vi "acquire waveform.vi"(0 "Connection ID":refnum<k5>, 5 "Server Stats":T1={"scan rate"=10.0, "# connections"=0, "channel settings"=[]} {"channel settings"."lower input limits" format="%.4f"; "channel settings"."upper input limits" format="%.4f"; "scan rate" format="%.2f"}, 7 "method":T2={"sampling interval"=0.1, "samples to average"=1, "data interval"=0.0, "stream data"=FALSE, "file path"=refnum, "command"={"command"=enum."Idle", "start time (ms)"=0, "Channel Indices"=[], "Scans per Sample"=1}} {"command"."Scans per Sample" min=1; "data interval" format="%.2f"; "samples to average" min=1 step=1; "sampling interval" format="%.2f"}, 11 "data points to acquire":u32=1000 min=1) -> (4 "data array":sgl[][](array[numeric]) format="%.5f", 6 "offset":sgl format="%.5f", 8 "percent CV":sgl format="%.5f")   [LabVIEW 2010]
uses:
  DataServer/command.ctl
  DataServer/command cluster.ctl
  DAC apps/support/method.ctl
  DataServer/Server stats.ctl
panel:
  in  "colors":u32[](array[colorbox])=[16711680, 13311, 52224, 16777215, 16750848, 16738047, 52479, 16776960, 16711680, 13311, 52224, 16777215, 16737792, 16738047, 52479, 16776960]
  out "sample time":dbl format="%.2f"
  out "stop":bool
  in  "State":cluster{"Monitor sample":bool, "Okay":bool}
  out "Scan rate":dbl=10.0
  out "data rate":sgl format="%.4f"
  out "sampling rate":dbl format="%.4f"
  out "chart":sgl[][](graph)
  in  "Monitoring sample":bool
  in  "error":errorcluster={"status"=FALSE, "code"=56, "source"="TCP Read in \u0000TCP read variable.vi->read Volts data fast.vi->Signal Monitor"}
  # "hz"
  # "hz"
  # "hz"
  # "s"
  # "Hz"
  # "s"
  # "s"
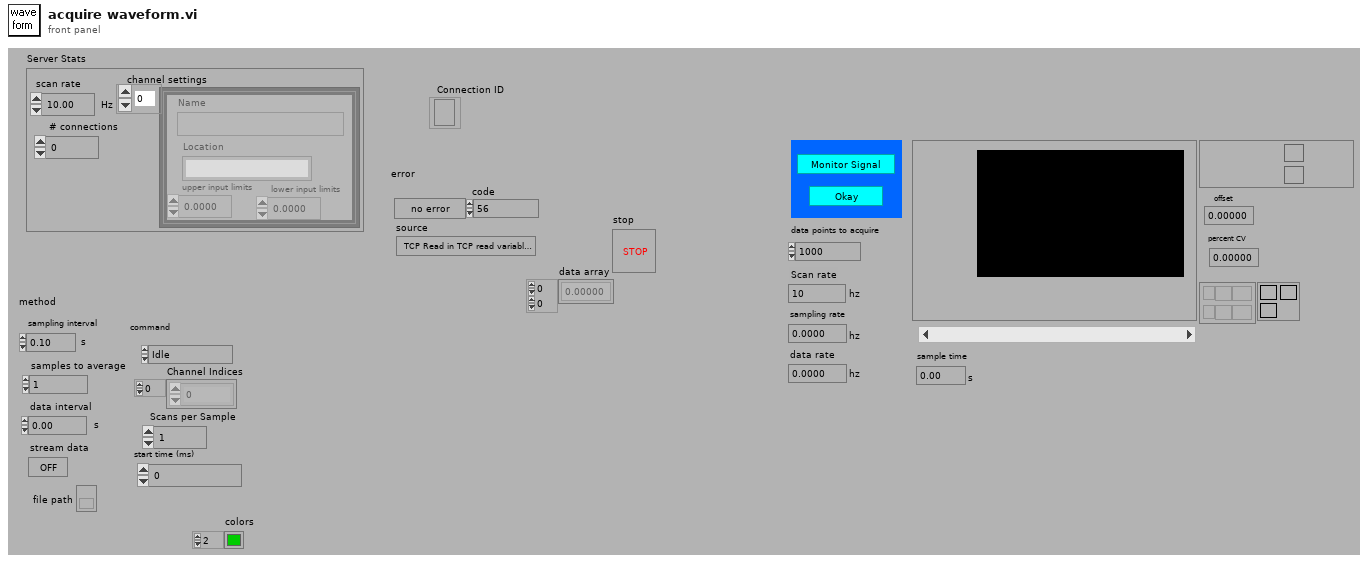
[diagram p1: front panel]
types:
  T1 = typedef "Server stats.ctl" = cluster{"scan rate":dbl, "# connections":i32, "channel settings":cluster{"Name":string, "upper input limits":sgl, "lower input limits":sgl, "Location":string}[]}
  T2 = typedef "method.ctl" = cluster{"sampling interval":sgl, "samples to average":u32, "data interval":sgl, "stream data":bool, "file path":refnum<file>, "command":T3}
  T3 = typedef "command cluster.ctl" = cluster{"command":T4, "start time (ms)":u32, "Channel Indices":i32[], "Scans per Sample":i32}
  T4 = typedef "command.ctl" = enum16{"Idle", "Send Data", "Send 1 Scan", "Logoff"}
  T5 = cluster{"channel":string, "upper input limits":sgl, "lower input limits":sgl, "range":sgl, "polarity":enum16{"no change", "bipolar", "unipolar"}, "gain":sgl, "coupling":enum16{"no change", "DC", "AC", "ground", "internal reference"}, "input mode":enum16{"no change", "differential", "rse", "nrse"}, "scale multiplier":sgl, "scale offset":sgl}[]
  T6 = cluster{"channel":string, "upper input limits":sgl, "lower input limits":sgl, "range":sgl, "polarity":enum16{"no change", "bipolar", "unipolar"}, "gain":sgl, "coupling":enum16{"no change", "DC", "AC", "ground", "internal reference"}, "input mode":enum16{"no change", "differential", "rse", "nrse"}, "scale multiplier":sgl, "scale offset":sgl}
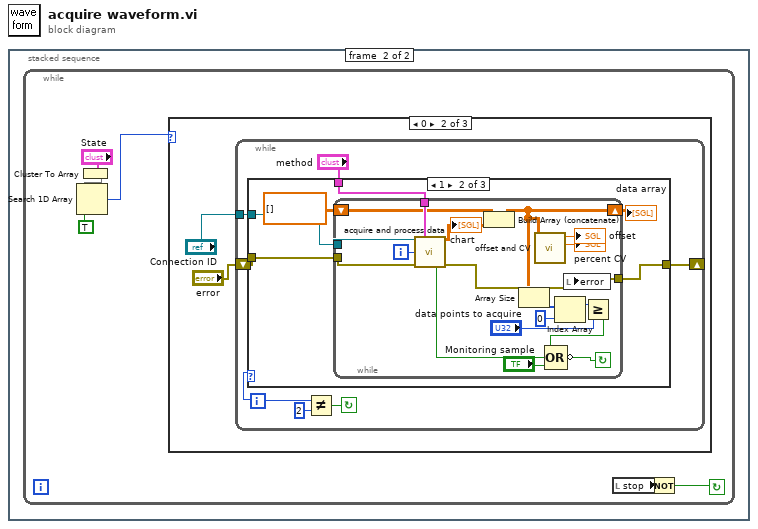
[diagram p0: block diagram]
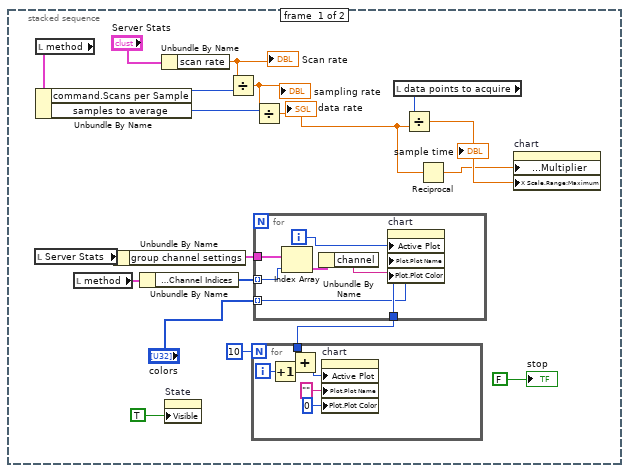
[diagram p2: hidden frame]
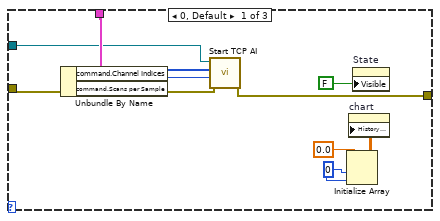
[diagram p4: hidden frame]
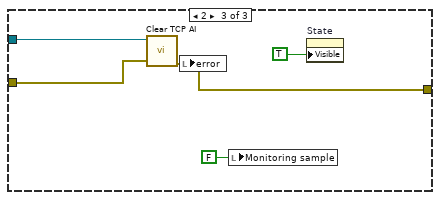
[diagram p5: hidden frame]
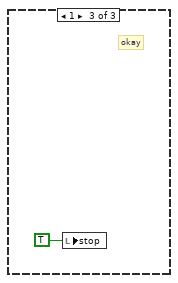
[diagram p6: hidden frame]
diagram:
  n1 = stacked-sequence {
    frame #0 {
      n2 = local read "Server Stats"() -> (w18:T1)
      n3 = local read "method"() -> (w2:T2)
      n4 = Unbundle By Name(w2) -> ("command.Scans per Sample"=w7:i32, "samples to average"=w8:u32)
      n5 = local read "method"() -> (w17:T2)
      n6 = Unbundle By Name(w18) -> ("group channel settings"=w15:T5)
      n7 = Unbundle By Name(w17) -> ("command.Channel Indices"=w16:i32[])
      n8 = Unbundle By Name("Server Stats") -> ("scan rate"=w10:dbl)
      "Scan rate" <- w10
      n9 = property on="State" class="Clust"("Visible"=TRUE ("Write Attribute")) -> ()  [unwired: 2 in, 2 out]
      n10 = Divide(x=w10, y=w7) -> (x/y=w9:dbl)
      "sampling rate" <- w9
      n11 = Divide(x=w9, y=w8) -> (x/y=w4:dbl)
      "data rate" <- w4
      n12 = for {
        tunnel: w16 -> [w31] mode=indexing
        tunnel: w15 -> [w30]
        tunnel: [w27] -> w13
        tunnel: "colors" -> [w26] mode=indexing
        i -> [w27]
        n13 = Index Array(array=w30, index=w31) -> (element=w29:T6)
        n14 = Unbundle By Name(w29) -> ("channel"=w28:string)
        n15 = property on="chart" class="WFChart (strict)"("Active Plot"=w27, "Plot.Plot Name"=w28, "Plot.Plot Color"=w26) -> ()  [unwired: 2 in, 2 out]
      }
      n16 = for {
        N: 10 -> [_]
        tunnel: w13 -> [w23]
        i -> [w25]
        n17 = Increment(x=w25) -> (x+1=w20:i32)
        n18 = Add(x=w23, y=w20) -> (x+y=w24:i32)
        n19 = property on="chart" class="WFChart (strict)"("Active Plot"=w24, "Plot.Plot Name"="" ("Write Attribute"), "Plot.Plot Color"=u32 0 ("Write Attribute")) -> ()  [unwired: 2 in, 2 out]
      }
      n20 = local read "data points to acquire"() -> (w6:u32)
      n21 = Divide(x=w6, y=w4) -> (x/y=w5:dbl)
      "sample time" <- w5
      n22 = Reciprocal(x=w4) -> (1/x=w3:dbl)
      n23 = property on="chart" class="WFChart (strict)"("X Scale.Offset and Multiplier:Multiplier"=w3, "X Scale.Range:Maximum"=w5) -> ()  [unwired: 2 in, 2 out]
      "stop" <- FALSE ("stop")
    }
    frame #1 {
      n24 = while {
        stop <- w32 continue-if-true
        n25 = Cluster To Array(cluster="State") -> (array=w37:bool[])
        n26 = Search 1D Array(1D array=w37, element=TRUE) -> (index of element=w34:i32)  [unwired: 1 in]
        n27 = case shown="0" w34 {
          frame -1, Default {
          }
          frame 0 {
            n28 = while {
              shift-left: "error" -> [w40]
              shift-right: [w41] -> _
              tunnel: "Connection ID" -> [w45]
              i -> [w44]
              stop <- w42 continue-if-true
              n29 = case shown="1" w44 {
                tunnel: [w48 w59 w81] -> w41
                tunnel: w40 -> [w47 w62 w82]
                tunnel: "method" -> [w56 w61 _]
                tunnel: w45 -> [w49 w60 w83]
                frame 0, Default {
                  w55 = 0
                  n30 = Unbundle By Name(w56) -> ("command.Channel Indices"=w50:i32[], "command.Scans per Sample"=w51:i32)
                  n31 = call "Start TCP AI.vi"("error in (no error)"=w47, "Scans per Sample"=w51, "channel indices"=w50, "Connection ID in"=w49) -> ("error out"=w48:errorcluster)  [unwired: 5 in, 2 out]
                  n32 = Initialize Array(sgl 0.0, w55, w55) -> (w53:sgl[][])
                  n33 = property on="chart" class="WFChart (strict)"("History Data"=w53) -> ()  [unwired: 2 in, 2 out]
                  n34 = property on="State" class="Clust"("Visible"=FALSE ("Write Attribute")) -> ()  [unwired: 2 in, 2 out]
                }
                frame 1 {
                  n35 = while {
                    shift-left: sgl[][] [] -> [w67]
                    shift-right: [w66] -> w58
                    tunnel: w60 -> [w73]
                    tunnel: w61 -> [w74]
                    tunnel: [w77] -> w59
                    tunnel: w62 -> [w76]
                    i -> [w63]
                    stop <- w80 continue-if-true
                    n36 = call "acquire and process data.vi"("connection ID"=w73, "Reset"=w63, "error in"=w76, "method"=w74) -> ("data out"=w78:sgl[][], "Status"=w75:bool, "error out"=w77:errorcluster)  [unwired: 4 in, 5 out]
                    "chart" <- w78
                    n37 = Build Array (concatenate)(w67, w78) -> (w66:sgl[][])
                    n38 = Array Size(array=w66) -> (size(s)=w72:i32[])
                    n39 = call "offset and CV.vi"("volts"=w66) -> ("percent CV"=→"percent CV":sgl, "mean"=→"offset":sgl)  [unwired: 9 in]
                    n40 = Index Array(array=w72, index=0 ("Index")) -> (element=w70:i32)
                    n41 = local write "error"(w77) -> ()
                    n42 = Greater Or Equal?(x=w70, y="data points to acquire") -> (x >= y?=w68:bool)
                    n43 = Compound Arithmetic op=OR(w68, w75, "Monitoring sample") -> (invert w80:bool)
                  }
                  "data array" <- w58
                }
                frame 2 {
                  n44 = call "Clear TCP AI.vi"("error in (no error)"=w82, "Connection ID in"=w83) -> ("error out"=w81:errorcluster)  [unwired: 8 in, 1 out]
                  n45 = local write "error"(w81) -> ()
                  n46 = local write "Monitoring sample"(FALSE ("Monitoring sample")) -> ()
                  n47 = property on="State" class="Clust"("Visible"=TRUE ("Write Attribute")) -> ()  [unwired: 2 in, 2 out]
                }
              }
              n48 = Not Equal?(x=w44, y=2) -> (x != y?=w42:bool)
            }
          }
          frame 1 {
            # "okay"
            n49 = local write "stop"(TRUE ("stop")) -> ()
          }
        }
        n50 = local read "stop"() -> (w33:bool)
        n51 = Not(x=w33) -> (.not. x?=w32:bool)
      }
    }
  }
